vi "Cal File Get Data In Range.vi"(9 "Requested Step Size":dbl, 10 "Data (sorted by frequency)":dbl[][](array[numeric]), 11 "Freq Sub-range":dbl[](array[numeric])) -> (2 "DATA Subset":dbl[][](array[numeric]))   [LabVIEW 2011]
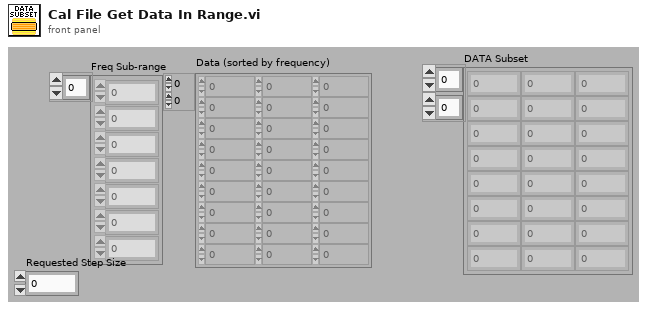
[diagram p1: front panel]
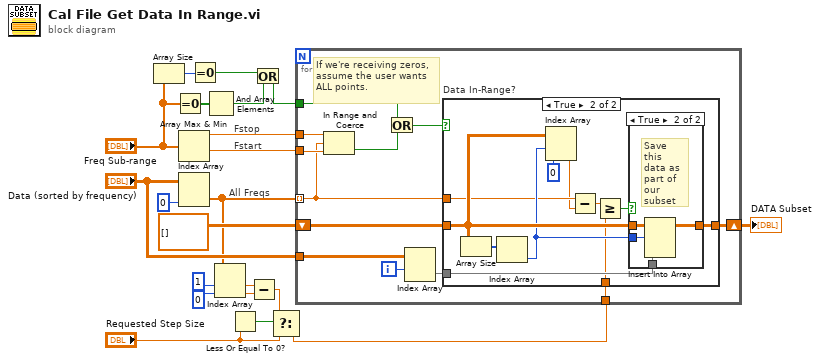
[diagram p0: block diagram]
diagram:
  # "Fstart"
  # "Fstop"
  # "All Freqs"
  n1 = Array Size(array="Freq Sub-range") -> (size(s)=w4:i32)
  n2 = Equal To 0?(x="Freq Sub-range") -> (x = 0?=w15:bool[])
  n3 = Array Max & Min(array="Freq Sub-range") -> (max value=w20:dbl, min value=w19:dbl)  [unwired: 2 out]
  n4 = Index Array(array="Data (sorted by frequency)", index (col)=0 ("disabled index (col)")) -> (element=w14:dbl[])  [unwired: 1 in]
  n5 = Equal To 0?(x=w4) -> (x = 0?=w3:bool)
  n6 = And Array Elements(Boolean array=w15) -> (logical AND=w2:bool)
  n7 = Index Array(array=w14, index #1=1 ("disabled index (col)"), index #2=0 ("disabled index (col)")) -> (element #1=w8:dbl, element #2=w7:dbl)
  n8 = Less Or Equal To 0?(x="Requested Step Size") -> (x <= 0?=w11:bool)
  n9 = Subtract(x=w8, y=w7) -> (x-y=w6:dbl)
  n10 = Or(x=w3, y=w2) -> (x .or. y?=w1:bool)
  n11 = Select(t=w6, s=w11, f="Requested Step Size") -> (s? t:f=w9:dbl)
  n12 = for {
    tunnel: w14 -> [w23] mode=indexing
    tunnel: w20 -> [w33]
    tunnel: w19 -> [w32]
    tunnel: "Data (sorted by frequency)" -> [w31]
    shift-right: [w28] -> w16
    shift-left: dbl[][] [] ("DATA @ FREQ") -> [w29]
    tunnel: w1 -> [w26]
    tunnel: w9 -> [w22]
    i -> [w30]
    # "If we're receiving zeros,\nassume the user wants\nALL points."
    n13 = In Range and Coerce(upper limit=w33, x=w23, lower limit=w32) -> (In Range?=w25:bool)  [unwired: 1 out]
    n14 = Or(x=w26, y=w25) -> (x .or. y?=w24:bool)
    n15 = Index Array(array=w31, index (row)=w30) -> (element=w27:dbl[])  [unwired: 1 in]
    n16 = case "Data In-Range?" shown="True" w24 {
      tunnel: w29 -> [w34 w42]
      tunnel: [w34 w43] -> w28
      tunnel: w27 -> [_ w45]
      tunnel: w23 -> [_ w39]
      tunnel: w22 -> [_ w36]
      frame False {
        # "Don't save this data"
      }
      frame True {
        n17 = Array Size(array=w42) -> (size(s)=w44:i32[])
        n18 = Index Array(array=w44) -> (element=w41:i32)  [unwired: 1 in]
        n19 = Index Array(array=w42, index (row)=w41, index (col)=0 ("disabled index (col)")) -> (element=w38:dbl)
        n20 = Subtract(x=w39, y=w38) -> (x-y=w37:dbl)
        n21 = Greater Or Equal?(x=w37, y=w36) -> (x >= y?=w35:bool)
        n22 = case shown="True" w35 {
          tunnel: w45 -> [_ w50]
          tunnel: [w46 w49] -> w43
          tunnel: w42 -> [w46 w48]
          tunnel: w41 -> [_ w47]
          frame False {
          }
          frame True {
            # "Save this data as part of our subset"
            n23 = Insert Into Array(array=w48, index (row)=w47, new element=w50) -> (w49:dbl[][])  [unwired: 1 in]
          }
        }
      }
    }
  }
  "DATA Subset" <- w16
